vi "Testing.vi"() -> ()   [LabVIEW 2021]
doc: "The myRIO Project template acquires acceleration data from the onboard accelerometer and displays the changes of acceleration values in a waveform chart."
uses:
  <vilib>/myRIO/Instrument Drivers/Onboard IO/DIO/typedefs/DIO Reference.ctl
  <vilib>/myRIO/Common/Instrument Driver Framework/Utilities/typedefs/myRIO Generic Hardware Reference.ctl
  <vilib>/myRIO/Common/Instrument Driver Framework/Utilities/typedefs/Hardware Version Enum.ctl
  <vilib>/myRIO/Common/Instrument Driver Framework/Utilities/typedefs/myRIO v1.0 Reference.ctl
  <vilib>/myRIO/Common/Instrument Driver Framework/Utilities/typedefs/Generic FPGA Reference.ctl
  <vilib>/myRIO/Common/Instrument Driver Framework/myRIO v1.0/DIO/typedefs/DIO Channels List.ctl
  <vilib>/myRIO/Common/Instrument Driver Framework/myRIO v1.0/DIO/typedefs/DIO Channels Enum.ctl
  <vilib>/userDefined/High Color/nirio_resource_hc.ctl
  <vilib>/myRIO/Instrument Drivers/Onboard IO/PWM/typedefs/PWM Reference.ctl
  <vilib>/myRIO/Common/Instrument Driver Framework/myRIO v1.0/PWM/typedefs/PWM Channels Enum.ctl
  <vilib>/myRIO/Instrument Drivers/Onboard IO/PWM/typedefs/PWM Configuration.ctl
  <vilib>/myRIO/Instrument Drivers/Onboard IO/AI/typedefs/AI Reference.ctl
  <vilib>/myRIO/Common/Instrument Driver Framework/myRIO v1.0/AI/typedefs/AI Channels List.ctl
  <vilib>/myRIO/Common/Instrument Driver Framework/myRIO v1.0/AI/typedefs/AI Channels Enum.ctl
  <vilib>/myRIO/Common/Instrument Driver Framework/Utilities/typedefs/Analog Scaling Constants List.ctl
  <vilib>/myRIO/Common/Instrument Driver Framework/Utilities/typedefs/Analog Scaling Constants.ctl
  <vilib>/myRIO/Common/Instrument Driver Framework/Utilities/vis/Is FPGA Ref Available.vi
  <vilib>/myRIO/Common/Instrument Driver Framework/myRIO v1.0/AI/vis/myRIO v1.1 Open AI.vi
  <vilib>/myRIO/Instrument Drivers/Onboard IO/AI/vis/Read.vi
  <vilib>/myRIO/Common/Instrument Driver Framework/myRIO v1.0/PWM/vis/myRIO v1.1 Open PWM.vi
  <vilib>/myRIO/Instrument Drivers/Onboard IO/PWM/vis/Set Duty Cycle and Frequency.vi
  <vilib>/myRIO/Common/Instrument Driver Framework/myRIO v1.0/DIO/vis/myRIO v1.1 Open DIO.vi
  <vilib>/myRIO/Instrument Drivers/Onboard IO/DIO/vis/Write.vi
  <vilib>/myRIO/Common/Instrument Driver Framework/Utilities/vis/Validate Channels.vi
  <vilib>/myRIO/Common/Instrument Driver Framework/myRIO v1.0/AI/vis/myRIO v1.0 Reserve AI.vi
  <vilib>/myRIO/Common/Instrument Driver Framework/myRIO v1.0/PWM/vis/myRIO v1.0 Reserve PWM.vi
  <vilib>/myRIO/Common/Instrument Driver Framework/myRIO v1.0/DIO/vis/myRIO v1.0 Reserve DIO.vi
  <vilib>/myRIO/Common/Instrument Driver Framework/myRIO v1.0/AI/vis/myRIO v1.0 Build MUX Configuration AI.vi
  <vilib>/myRIO/Common/Instrument Driver Framework/myRIO v1.0/Resource Manager/vis/myRIO v1.0 Reserve Channel List.vi
  <vilib>/myRIO/Common/Instrument Driver Framework/myRIO v1.0/PWM/vis/myRIO v1.0 Build MUX Configuration PWM.vi
  <vilib>/myRIO/Common/Instrument Driver Framework/myRIO v1.0/DIO/vis/myRIO v1.0 Build MUX Configuration DIO.vi
  <vilib>/myRIO/Common/Instrument Driver Framework/myRIO v1.0/Resource Manager/vis/myRIO v1.0 Reserve Channel.vi
  <vilib>/myRIO/Common/Instrument Driver Framework/myRIO v1.0/Resource Manager/vis/myRIO v1.0 Unreserve Channel.vi
  <vilib>/myRIO/Common/Instrument Driver Framework/myRIO v1.0/Resource Manager/vis/myRIO v1.0 Create Configuration List.vi
  <vilib>/myRIO/Common/Instrument Driver Framework/myRIO v1.0/Resource Manager/vis/myRIO v1.0 Build Mutex Name.vi
  <vilib>/addons/control/pid/pid.llb/PID (DBL).vi
  <vilib>/Utility/VariantDataType/GetNumericInfo.vi
  <vilib>/Utility/error.llb/Error Cluster From Error Code.vi
  <vilib>/myRIO/Common/Instrument Driver Framework/myRIO v1.0/myRIO v1.1 Open.vi
  <vilib>/myRIO/Common/Instrument Driver Framework/Utilities/vis/IO Manager.vi
  <vilib>/myRIO/Common/Instrument Driver Framework/Utilities/vis/Configuration Manager.vi
  <vilib>/myRIO/Common/Instrument Driver Framework/myRIO v1.0/Resource Manager/vis/myRIO v1.0 Configure IO.vi
  <vilib>/myRIO/Common/Instrument Driver Framework/myRIO v1.0/myRIO v1.0 Close.vi
  <vilib>/myRIO/Common/Instrument Driver Framework/myRIO v1.0/DIO/vis/myRIO v1.0 Write DIO.vi
  <vilib>/myRIO/Common/Instrument Driver Framework/myRIO v1.0/PWM/vis/myRIO v1.0 Write PWM.vi
  <vilib>/myRIO/Common/Instrument Driver Framework/myRIO v1.0/AI/vis/myRIO v1.0 Get Scaling Constants AI.vi
  <vilib>/myRIO/Common/Instrument Driver Framework/myRIO v1.0/AI/vis/myRIO v1.0 Read AI.vi
  <vilib>/myRIO/Express VI/Onboard IO/DO/DO Express VI.xnode
  <vilib>/myRIO/Instrument Drivers/Onboard IO/DIO/vis/myRIO DIO Open.xnode
  <vilib>/myRIO/Express VI/Onboard IO/PWM/PWM Express VI.xnode
  <vilib>/myRIO/Instrument Drivers/Onboard IO/PWM/vis/myRIO PWM Open.xnode
  <vilib>/myRIO/Express VI/Onboard IO/AI/AI Express VI.xnode
  <vilib>/myRIO/Instrument Drivers/Onboard IO/AI/vis/myRIO AI Open.xnode
  <vilib>/myRIO/Instrument Drivers/Onboard IO/DIO/DIO.lvlib
  <vilib>/myRIO/Instrument Drivers/Onboard IO/AI/AI.lvlib
  <vilib>/addons/control/pid/NI_PID_pid.lvlib
  <vilib>/myRIO/Instrument Drivers/Onboard IO/PWM/PWM.lvlib
panel:
  in  "Home Position":dbl=250.0
  out "Elapsed Time":dbl
  out "Run Motor PWM":dbl
  out "Initialise Motor PWM":dbl
  in  "Drop-Off Angle":dbl=90.0
  out "Drop-Off Position":dbl
  out "Complete Stop Position":dbl
  in  "Complete Stop Angle":dbl=45.0
  in  "Manual Mode switch":bool
  in  "DIO4":bool
  in  "DIO5":bool
  in  "DIO6":bool
  in  "DIO7":bool
  in  "PID Gains":T1={"Proportional Gain, Kc"=0.5, "Integral Time, ti"=0.1, "Derivative Time, td"=0.1}
  out "Angle":dbl
  out "AI3":dbl
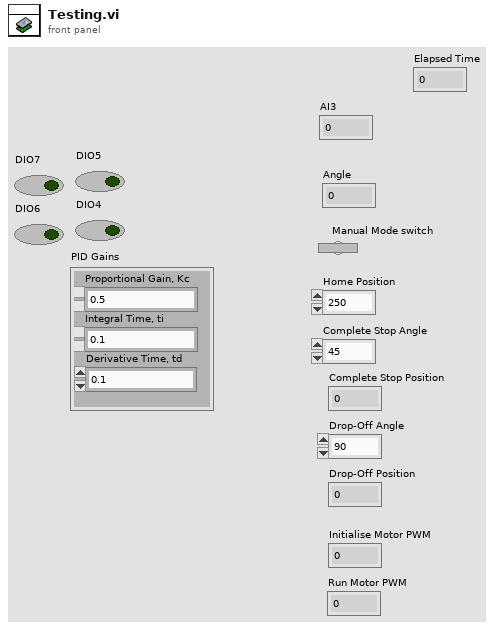
[diagram p1: front panel]
types:
  T1 = cluster{"Proportional Gain, Kc":dbl, "Integral Time, ti":dbl, "Derivative Time, td":dbl}
  T2 = typedef "AI.lvlib/AI Reference.ctl" = cluster{"myRIO Reference":T3, "AI Channels List":T7, "AI Scaling Constants List":T9}
  T3 = typedef "myRIO Generic Hardware Reference.ctl" = cluster{"myRIO Model":T4, "myRIO Hardware Reference":T5}
  T4 = typedef "Hardware Version Enum.ctl" = enum16{"Unknown", "myRIO-1900", "myRIO-1950", "roboRIO", "NI ELVIS RIO CM", "ELVIS III"}
  T5 = typedef "myRIO v1.0 Reference.ctl" = cluster{"Generic FPGA Reference":T6, "Allow multiple opens":bool}
  T6 = typedef "Generic FPGA Reference.ctl" = refnum<k20>
  T7 = typedef "AI Channels List.ctl" = T8[]
  T8 = typedef "AI Channels Enum.ctl" = enum16{"Not Connected", "AudioIn/Left", "AudioIn/Right", "C/AI0", "C/AI1", "A/AI0", "A/AI1", "A/AI2", "A/AI3", "A/AI4", "A/AI5", "A/AI6", "A/AI7", "B/AI0", "B/AI1", "B/AI2", "B/AI3", "B/AI4", "B/AI5", "B/AI6", "B/AI7", "AI/AI0", "AI/AI1", "AI/AI2", "AI/AI3", "A/AI0 (DIFF)", "A/AI1 (DIFF)", "A/AI2 (DIFF)", "A/AI3 (DIFF)", "B/AI0 (DIFF)", "B/AI1 (DIFF)", "B/AI2 (DIFF)", "B/AI3 (DIFF)"}
  T9 = typedef "Analog Scaling Constants List.ctl" = T10[]
  T10 = typedef "Analog Scaling Constants.ctl" = cluster{"LSB Weight (Volts)":dbl, "Offset (Volts)":dbl, "Signed?":bool}
  T11 = typedef "nirio_resource_hc.ctl" = tag
  T12 = typedef "DIO.lvlib/DIO Reference.ctl" = cluster{"myRIO Reference":T3, "DIO Channels List":T13}
  T13 = typedef "DIO Channels List.ctl" = T14[]
  T14 = typedef "DIO Channels Enum.ctl" = enum16{"Not Connected", "C/DIO0", "C/DIO1", "C/DIO2", "C/DIO3", "C/DIO4", "C/DIO5", "C/DIO6", "C/DIO7", "A/DIO0", "A/DIO1", "A/DIO2", "A/DIO3", "A/DIO4", "A/DIO5", "A/DIO6", "A/DIO7", "A/DIO8", "A/DIO9", "A/DIO10", "A/DIO11", "A/DIO12", "A/DIO13", "A/DIO14", "A/DIO15", "A/DIO16", "A/DIO17", "A/DIO18", "A/DIO19", "B/DIO0", "B/DIO1", "B/DIO2", "B/DIO3", "B/DIO4", "B/DIO5", "B/DIO6", "B/DIO7", "B/DIO8", "B/DIO9", "B/DIO10", "B/DIO11", "B/DIO12", "B/DIO13", "B/DIO14", "B/DIO15", "B/DIO16", "B/DIO17", "B/DIO18", "B/DIO19", "LED0", "LED1", "LED2", "LED3", "Button0", "DIO/DIO0", "DIO/DIO1", "DIO/DIO2", "DIO/DIO3", "DIO/DIO4", "DIO/DIO5", "DIO/DIO6", "DIO/DIO7", "DIO/DIO8", "DIO/DIO9", "SPI/CS0", "SPI/CS1", "SPI/CS2", "SPI/CS3", "LED RADIO (Green)", "LED RADIO (Red)", "LED COMM (Green)", "LED COMM (Red)", "LED MODE (Green)", "LED MODE (Red)"}
  T15 = typedef "PWM.lvlib/PWM Reference.ctl" = cluster{"myRIO Reference":T3, "PWM Channels Enum":T16, "PWM Configuration":T17}
  T16 = typedef "PWM Channels Enum.ctl" = enum16{"Not Connected", "C/PWM0", "C/PWM1", "A/PWM0", "A/PWM1", "A/PWM2", "A/PWM3", "A/PWM4", "A/PWM5", "A/PWM6", "A/PWM7", "A/PWM8", "A/PWM9", "A/PWM10", "A/PWM11", "A/PWM12", "A/PWM13", "A/PWM14", "A/PWM15", "A/PWM16", "A/PWM17", "A/PWM18", "A/PWM19", "B/PWM0", "B/PWM1", "B/PWM2", "B/PWM3", "B/PWM4", "B/PWM5", "B/PWM6", "B/PWM7", "B/PWM8", "B/PWM9", "B/PWM10", "B/PWM11", "B/PWM12", "B/PWM13", "B/PWM14", "B/PWM15", "B/PWM16", "B/PWM17", "B/PWM18", "B/PWM19", "PWM/PWM0", "PWM/PWM1", "PWM/PWM2", "PWM/PWM3", "PWM/PWM4", "PWM/PWM5", "PWM/PWM6", "PWM/PWM7", "PWM/PWM8", "PWM/PWM9"}
  T17 = typedef "PWM.lvlib/PWM Configuration.ctl" = cluster{"Frequency":dbl, "Duty Cycle":dbl}
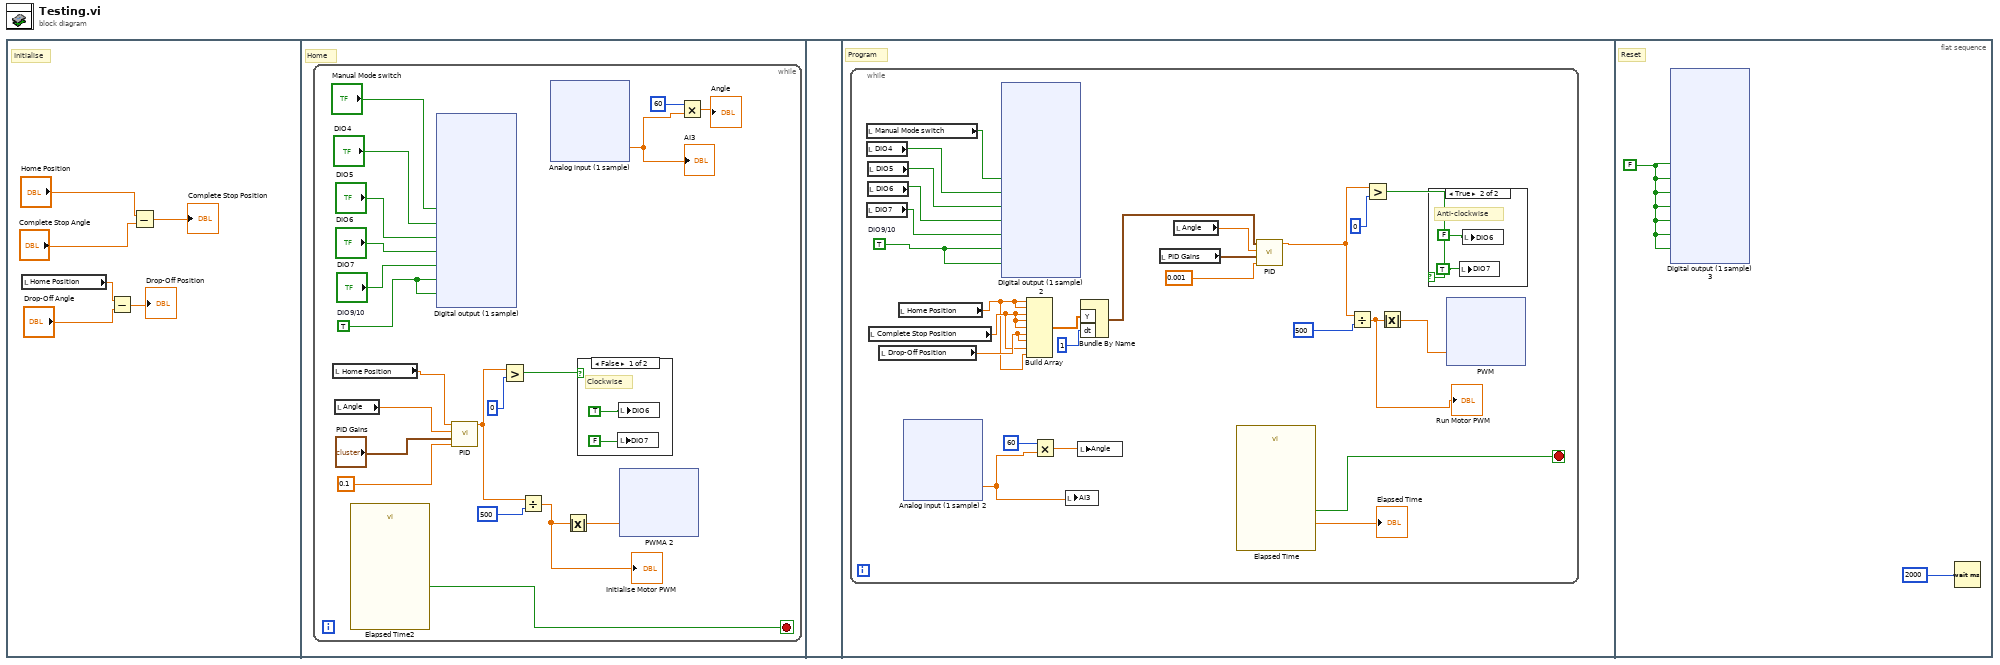
[diagram p0: block diagram]
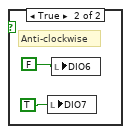
[diagram p2: hidden frame]
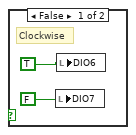
[diagram p3: hidden frame]
diagram:
  n1 = flat-sequence {
    frame #0 {
      # "Initialise"
      n2 = local read "Home Position"() -> (w4:dbl)
      n3 = Subtract(x=w4, y="Drop-Off Angle") -> (x-y=→"Drop-Off Position":dbl)
      n4 = Subtract(x="Home Position", y="Complete Stop Angle") -> (x-y=→"Complete Stop Position":dbl)
    }
    frame #1 {
      # "Home"
      n5 = while {
        stop <- w7 stop-if-true
        w11 = TRUE  # DIO9/10
        n6 = local read "Home Position"() -> (w8:dbl)
        n7 = local read "Angle"() -> (w20:dbl)
        n8 = call "Elapsed Time2"() -> ("Time has Elapsed"=w7:bool)  [unwired: 12 in, 7 out]
        n9 = xnode "Digital output (1 sample)"("Auto/Manual Mode Switch (A/DIO3 (Pin 17))"="Manual Mode switch", "Solenoid 1 (A/DIO4 (Pin 19))"="DIO4", "Solenoid 2 (A/DIO5 (Pin 21))"="DIO5", "Motor Clockwise (A/DIO6 (Pin 23))"="DIO6", "Motor Anti-Clockwise (A/DIO7 (Pin 25))"="DIO7", "Solenoid PWM (A/DIO9 (Pin 29))"=w11, "Motor Driver Chip Standby (A/DIO10 (Pin 31))"=w11) -> ()  [unwired: 1 in, 1 out]
        n10 = call-poly <vilib>:"PID.vi"("dt (s)"=0.1, "PID gains"="PID Gains", "process variable"=w20, "setpoint"=w8) -> ("output"=w22:dbl)  [unwired: 6 in, 1 out]
        n11 = Greater?(x=w22, y=0) -> (0:w24:bool)
        n12 = Divide(x=w22, y=500) -> (x/y=w9:dbl)
        "Initialise Motor PWM" <- w9
        n13 = xnode "Analog input (1 sample)"() -> ("Motor Position (A/AI3 (Pin 9))"=w10:dbl)  [unwired: 1 in, 1 out]
        "AI3" <- w10
        n14 = Absolute Value(x=w9) -> (abs(x)=w17:dbl)
        n15 = case shown="False" w24 {
          frame False {
            # "Clockwise"
            n16 = local write "DIO7"(FALSE) -> ()
            n17 = local write "DIO6"(TRUE) -> ()
          }
          frame True {
            # "Anti-clockwise"
            n18 = local write "DIO7"(TRUE) -> ()
            n19 = local write "DIO6"(FALSE) -> ()
          }
        }
        n20 = xnode "PWMA 2"("Duty Cycle"=w17) -> ()  [unwired: 1 in, 1 out]
        n21 = Multiply(x=60, y=w10) -> (x*y=→"Angle":dbl)
      }
    }
    frame #2 {
    }
    frame #3 {
      # "Program"
      n22 = while {
        stop <- w148 stop-if-true
        w151 = TRUE  # DIO9/10
        n23 = local read "Manual Mode switch"() -> (w156:bool)
        n24 = local read "DIO4"() -> (w155:bool)
        n25 = local read "DIO7"() -> (w152:bool)
        n26 = local read "DIO5"() -> (w154:bool)
        n27 = local read "DIO6"() -> (w153:bool)
        n28 = local read "Complete Stop Position"() -> (w160:dbl)
        n29 = local read "Drop-Off Position"() -> (w162:dbl)
        n30 = local read "Home Position"() -> (w159:dbl)
        n31 = xnode "Analog input (1 sample) 2"() -> ("Motor Position (A/AI3 (Pin 9))"=w145:dbl)  [unwired: 1 in, 1 out]
        n32 = xnode "Digital output (1 sample) 2"("Auto/Manual Mode Switch (A/DIO3 (Pin 17))"=w156, "Solenoid 1 (A/DIO4 (Pin 19))"=w155, "Solenoid 2 (A/DIO5 (Pin 21))"=w154, "Motor Clockwise (A/DIO6 (Pin 23))"=w153, "Motor Anti-Clockwise (A/DIO7 (Pin 25))"=w152, "Solenoid PWM (A/DIO9 (Pin 29))"=w151, "Motor Driver Chip Standby (A/DIO10 (Pin 31))"=w151) -> ()  [unwired: 1 in, 1 out]
        n33 = Build Array(w159, w159, w160, w160, w160, w162, w162, w160, w159) -> (w163:dbl[])
        n34 = Multiply(x=60, y=w145) -> (x*y=w146:dbl)
        n35 = local write "AI3"(w145) -> ()
        n36 = local write "Angle"(w146) -> ()
        n37 = Bundle By Name("Y"=w163, "dt"=1) -> (w144:waveform(dbl))  [unwired: 1 in]
        n38 = local read "PID Gains"() -> (w164:T1)
        n39 = local read "Angle"() -> (w169:dbl)
        n40 = call "Elapsed Time"() -> ("Elapsed Time (s)"=→"Elapsed Time":dbl, "Time has Elapsed"=w148:bool)  [unwired: 12 in, 6 out]
        n41 = call-poly <vilib>:"PID.vi"("dt (s)"=0.001, "PID gains"=w164, "process variable"=w169, "setpoint"=w144) -> ("output"=w158:dbl)  [unwired: 6 in, 1 out]
        n42 = Divide(x=w158, y=500) -> (x/y=w150:dbl)
        "Run Motor PWM" <- w150
        n43 = Greater?(x=w158, y=0) -> (0:w167:bool)
        n44 = Absolute Value(x=w150) -> (abs(x)=w157:dbl)
        n45 = case shown="True" w167 {
          frame False {
            # "Clockwise"
            n46 = local write "DIO7"(FALSE) -> ()
            n47 = local write "DIO6"(TRUE) -> ()
          }
          frame True {
            # "Anti-clockwise"
            n48 = local write "DIO7"(TRUE) -> ()
            n49 = local write "DIO6"(FALSE) -> ()
          }
        }
        n50 = xnode "PWM"("Duty Cycle"=w157) -> ()  [unwired: 1 in, 1 out]
      }
    }
    frame #4 {
      w287 = FALSE
      # "Reset"
      n51 = xnode "Digital output (1 sample) 3"("Auto/Manual Mode Switch (A/DIO3 (Pin 17))"=w287, "Solenoid 1 (A/DIO4 (Pin 19))"=w287, "Solenoid 2 (A/DIO5 (Pin 21))"=w287, "Motor Clockwise (A/DIO6 (Pin 23))"=w287, "Motor Anti-Clockwise (A/DIO7 (Pin 25))"=w287, "Solenoid PWM (A/DIO9 (Pin 29))"=w287, "Motor Driver Chip Standby (A/DIO10 (Pin 31))"=w287) -> ()  [unwired: 1 in, 1 out]
      n52 = Wait (ms)(milliseconds to wait=2000) -> ()  [unwired: 1 out]
    }
  }
